vi "בדיקת מתח שחרור של סליל פיקוד ללא עומס 4.vi"(7 "resultUserPrompt":bool=TRUE, 8 "error":errorcluster, 11 "Path for Log":path) -> (0 "error out":errorcluster, 1 "מצב ממסר פתוח/סגור":bool, 2 "מתח פתיחת הממסר":dbl format="%.4f", 3 "מתח מוצא מהספק":dbl format="%.4f")   [LabVIEW 2015]
uses:
  <vilib>/DAQmx/write.llb/DAQmx Write (Digital Bool 1Line 1Point).vi
  <vilib>/DAQmx/create/channels.llb/DAQmx Create Channel (DO-Digital Output).vi
  <vilib>/DAQmx/miscellaneous.llb/DAQmx Fill In Error Info.vi
panel:
  out "progress":dbl(slide) scale=0.0..11.0
  out "error IO DMM":errorcluster
  in  "Stop Button":bool
  # "Right-Click to\nexplain error"
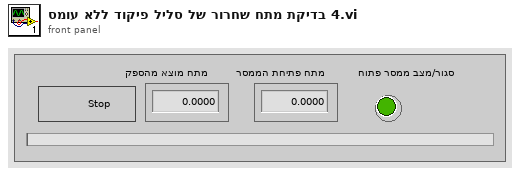
[diagram p1: front panel]
types:
  T1 = enum32{"Invalid", "Standard", "Closed", "Hidden", "Minimized", "Maximized"}
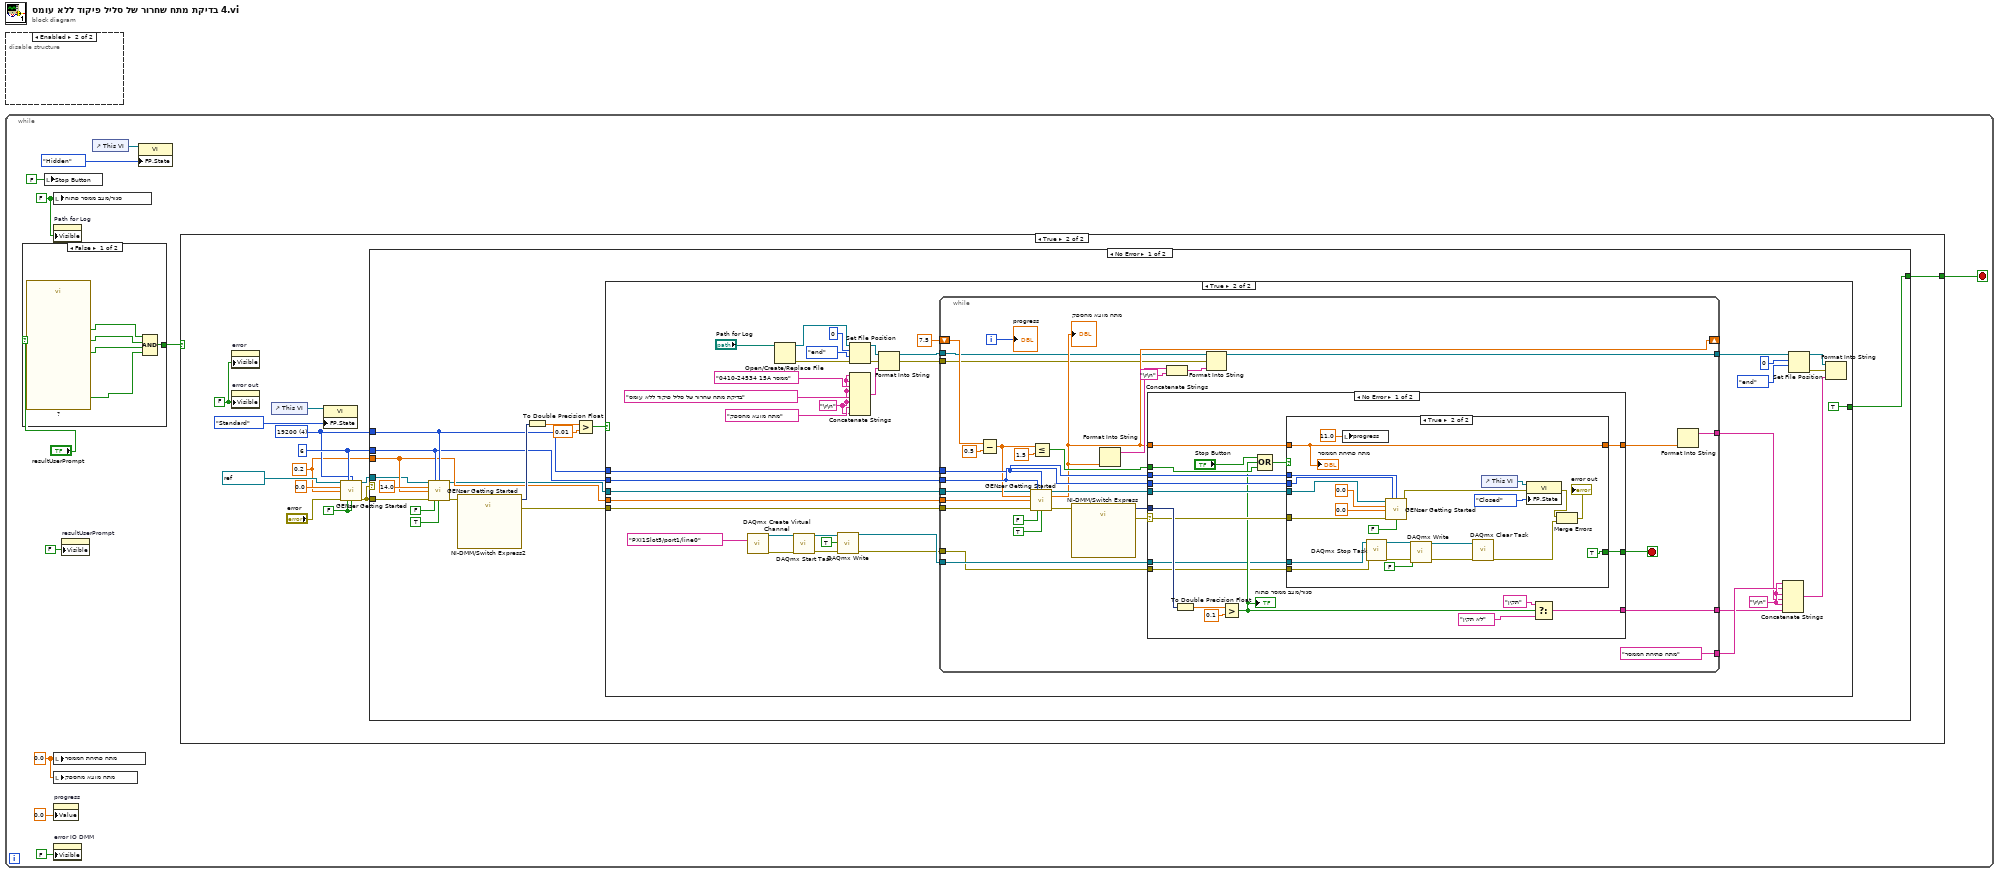
[diagram p0: block diagram]
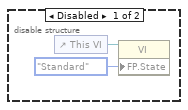
[diagram p2: hidden frame]
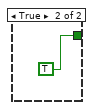
[diagram p3: hidden frame]
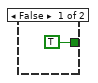
[diagram p4: hidden frame]
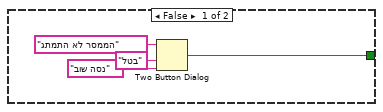
[diagram p5: hidden frame]
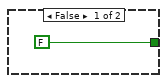
[diagram p6: hidden frame]
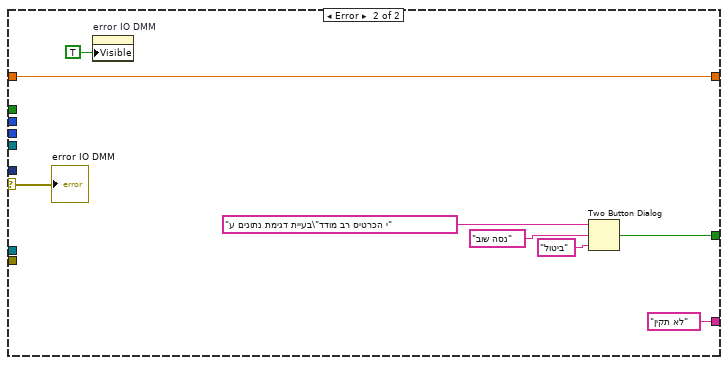
[diagram p7: hidden frame]
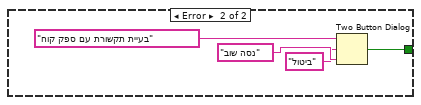
[diagram p8: hidden frame]
diagram:
  n1 = disable-structure shown="Enabled" {
    frame Disabled {
      n2 = control-ref of="This VI"() -> (w1:refnum<vi>)
      n3 = property class="VI"(reference=w1, "FP.State"=T1."Standard" ("Front Panel Window:State")) -> ()  [unwired: 1 in, 2 out]
    }
    frame Enabled {
    }
  }
  n4 = while {
    stop <- w3 stop-if-true
    w7 = FALSE ("מגע סגור")
    w10 = 0.0 ("signals out")
    n5 = case shown="False" "resultUserPrompt" {
      tunnel: [w18 TRUE] -> w4
      frame False {
        n6 = call "?"() -> ("הדקי הרב מודד"=w14:bool, "(מגע שלילי (מעטפת"=w15:bool, "A מגע חיובי"=w16:bool, "OK"=w17:bool)  [unwired: 15 in, 1 out]
        n7 = Compound Arithmetic op=AND(w17, w16, w15, w14) -> (w18:bool)
      }
      frame True {
      }
    }
    n8 = local write "Stop Button"(FALSE ("Reset (T)")) -> ()
    n9 = local write "מצב ממסר פתוח/סגור"(w7) -> ()
    n10 = property on="Path for Log" class="Path"("Visible"=w7) -> ()  [unwired: 2 in, 2 out]
    n11 = local write "מתח פתיחת הממסר"(w10) -> ()
    n12 = local write "מתח מוצא מהספק"(w10) -> ()
    n13 = property on="progress" class="Slide (strict)"("Value"=0.0 ("progress")) -> ()  [unwired: 2 in, 2 out]
    n14 = property on="error IO DMM" class="Clust (strict)"("Visible"=FALSE) -> ()  [unwired: 2 in, 2 out]
    n15 = property on="resultUserPrompt" class="Bool (strict)"("Visible"=FALSE) -> ()  [unwired: 2 in, 2 out]
    n16 = control-ref of="This VI"() -> (w9:refnum<vi>)
    n17 = property class="VI"(reference=w9, "FP.State"=T1."Hidden" ("Front Panel Window:State")) -> ()  [unwired: 1 in, 2 out]
    n18 = case shown="True" w4 {
      tunnel: [TRUE ("T button?") w25] -> w3
      frame False {
      }
      frame True {
        w23 = FALSE ("Visible")
        w24 = FALSE ("Output On (T)")
        w29 = u16 4 items=["1200", "2400", "4800", "9600", "19200"] ("BAUD")
        w30 = i16 6 ("GEN Addr")
        w26 = 0.2 ("Current Limit")
        n19 = property on="error" class="Clust (strict)"("Visible"=w23) -> ()  [unwired: 2 in, 2 out]
        n20 = property on="error out" class="Clust (strict)"("Visible"=w23) -> ()  [unwired: 2 in, 2 out]
        n21 = control-ref of="This VI"() -> (w21:refnum<vi>)
        n22 = property class="VI"(reference=w21, "FP.State"=T1."Standard" ("Front Panel Window:State")) -> ()  [unwired: 1 in, 2 out]
        n23 = call "GENser Getting Started.vi"("VISA"=refnum<visa-resource-name> "COM6", "GEN Addr"=w30, "BAUD"=w29, "Voltage Limit"=0.0, "Current Limit"=w26, "error"="error", "Reset (T)"=w24, "Output On (T)"=w24) -> ("VISA out"=w31:refnum<visa-resource-name>, "error out"=w32:errorcluster)  [unwired: 4 in, 2 out]
        n24 = case shown="No Error" w32 {
          tunnel: w32 -> [w42 _]
          tunnel: w31 -> [w38 _]
          tunnel: w30 -> [w40 _]
          tunnel: w29 -> [w41 _]
          tunnel: w26 -> [w39 _]
          tunnel: [w34 w177] -> w25
          frame No Error {
            n25 = call "GENser Getting Started.vi"("VISA"=w38, "GEN Addr"=w40, "BAUD"=w41, "Voltage Limit"=14.0, "Current Limit"=w39, "error"=w42, "Reset (T)"=FALSE, "Output On (T)"=TRUE) -> ("VISA out"=w37:refnum<visa-resource-name>, "error out"=w46:errorcluster)  [unwired: 4 in, 2 out]
            n26 = call "NI-DMM/Switch Express2"("error in"=w46) -> ("signals out"=w45:dynamicdata, "error out"=w43:errorcluster)  [unwired: 16 in, 1 out]
            n27 = To Double Precision Float(number=w45) -> (double precision float=w36:dbl)
            n28 = Greater?(x=w36, y=0.01) -> (0:w44:bool)
            n29 = case shown="True" w44 {
              tunnel: w43 -> [_ w92]
              tunnel: w40 -> [_ w91]
              tunnel: w41 -> [_ w90]
              tunnel: w39 -> [_ w89]
              tunnel: w37 -> [_ w87]
              tunnel: [w50 TRUE] -> w34
              frame False {
                n30 = Two Button Dialog(message="הממסר לא התמתג", 1:"נסה שוב" ("T button name (\"OK\")"), 2:"בטל" ("T button name (\"OK\")")) -> (T button?=w50:bool)
              }
              frame True {
                w63 = "\r\n"
                w86 = "\r\n"
                n31 = call-poly <vilib>:"DAQmx Create Virtual Channel.vi"("lines"=tag "PXI1Slot5/port1/line0") -> ("task out"=w61:refnum<k21>, "error out"=w62:errorcluster)  [unwired: 13 in]
                n32 = Open/Create/Replace File(file path (use dialog)="Path for Log") -> (refnum out=w74:refnum<file>, error out=w73:errorcluster)  [unwired: 5 in, 1 out]
                n33 = call <vilib>:"DAQmx Start Task.vi"("task/channels in"=w61, "error in"=w62) -> ("task out"=w59:refnum<k21>, "error out"=w58:errorcluster)  [unwired: 12 in]
                n34 = call-poly <vilib>:"DAQmx Write.vi"("task/channels in"=w59, "data"=TRUE, "error in"=w58) -> ("task out"=w56:refnum<k21>, "error out"=w55:errorcluster)  [unwired: 10 in, 1 out]
                n35 = Set File Position(offset (in bytes) (0)=i64 0, refnum=w74, from (0:start)=enum16{"start", "end", "current"}."end", error in=w73) -> (refnum out=w69:refnum<file>, error out=w64:errorcluster)
                n36 = Concatenate Strings(w63, w63, "0410-24534 15A ממסר", w63, "בדיקת מתח שחרור של סליל פיקוד ללא עומס", w63, "מתח מוצא מהספק", w63) -> (w72:string)
                n37 = Format Into String(initial string=w69, error in=w64, w72) -> (resulting string=w66:refnum<file>, error out=w65:errorcluster)  [unwired: 1 in]
                n38 = while {
                  tunnel: w92 -> [w123]
                  tunnel: w91 -> [w115]
                  tunnel: w90 -> [w114]
                  tunnel: w89 -> [w121]
                  shift-right: [w97] -> _
                  shift-left: 7.5 ("y") -> [w119]
                  tunnel: w87 -> [w107]
                  tunnel: [w102] -> w81
                  tunnel: ["מתח פתיחת הממסר"] -> w80
                  tunnel: [w100] -> w79
                  tunnel: [w99] -> w78
                  tunnel: w66 -> [w96]
                  tunnel: w65 -> [w95]
                  tunnel: w56 -> [w94]
                  tunnel: w55 -> [w93]
                  i -> [w108]
                  stop <- w116 stop-if-true
                  n39 = Subtract(x=w119, y=0.5) -> (x-y=w111:dbl)
                  n40 = call "GENser Getting Started.vi"("VISA"=w107, "GEN Addr"=w115, "BAUD"=w114, "Voltage Limit"=w111, "Current Limit"=w121, "error"=w123, "Reset (T)"=FALSE, "Output On (T)"=TRUE) -> ("VISA out"=w113:refnum<visa-resource-name>, "Output Voltage"=w97:dbl, "error out"=w118:errorcluster)  [unwired: 4 in, 1 out]
                  "מתח מוצא מהספק" <- w97
                  n41 = Less Or Equal?(x=w111, y=1.5) -> (x <= y?=w110:bool)
                  n42 = call "NI-DMM/Switch Express"("error in"=w118) -> ("signals out"=w117:dynamicdata, "error out"=w109:errorcluster)  [unwired: 16 in, 1 out]
                  n43 = Format Into String(w97) -> (resulting string=w104:string)  [unwired: 3 in, 1 out]
                  n44 = case shown="No Error" w109 {
                    selector: w109 -> [w133 w174]
                    tunnel: w117 -> [w142 _]
                    tunnel: [w139 w170] -> w116
                    tunnel: w115 -> [w138 _]
                    tunnel: w114 -> [w137 _]
                    tunnel: w113 -> [w136 _]
                    tunnel: w110 -> [w135 _]
                    tunnel: w97 -> [w134 w168]
                    tunnel: [w127 w168] -> w103
                    tunnel: [w126 "לא תקין"] -> w99
                    tunnel: w94 -> [w125 _]
                    tunnel: w93 -> [w124 _]
                    frame No Error {
                      n45 = To Double Precision Float(number=w142) -> (double precision float=w132:dbl)
                      n46 = Greater?(x=w132, y=0.1) -> (0:w128:bool)
                      "מצב ממסר פתוח/סגור" <- w128
                      n47 = Compound Arithmetic op=OR("Stop Button", w128, w135) -> (w141:bool)
                      n48 = case shown="True" w141 {
                        tunnel: [FALSE TRUE] -> w139
                        tunnel: w138 -> [_ w165]
                        tunnel: w137 -> [_ w164]
                        tunnel: w136 -> [_ w163]
                        tunnel: w133 -> [_ w160]
                        tunnel: w134 -> [_ w154]
                        tunnel: [_ w154] -> w127
                        tunnel: w125 -> [_ w148]
                        tunnel: w124 -> [_ w147]
                        frame False {
                        }
                        frame True {
                          n49 = local write "progress"(11.0 ("progress")) -> ()
                          n50 = call <vilib>:"DAQmx Stop Task.vi"("task/channels in"=w148, "error in"=w147) -> ("task out"=w153:refnum<k21>, "error out"=w152:errorcluster)  [unwired: 12 in]
                          n51 = call "GENser Getting Started.vi"("VISA"=w163, "GEN Addr"=w165, "BAUD"=w164, "Voltage Limit"=0.0, "Current Limit"=0.0, "error"=w160, "Output On (T)"=FALSE) -> ("error out"=w155:errorcluster)  [unwired: 5 in, 3 out]
                          n52 = call-poly <vilib>:"DAQmx Write.vi"("task/channels in"=w153, "data"=FALSE, "error in"=w152) -> ("task out"=w151:refnum<k21>, "error out"=w150:errorcluster)  [unwired: 10 in, 1 out]
                          n53 = call <vilib>:"DAQmx Clear Task.vi"("task in"=w151, "error in"=w150) -> ("error out"=w146:errorcluster)  [unwired: 13 in]
                          n54 = control-ref of="This VI"() -> (w156:refnum<vi>)
                          n55 = property class="VI"(reference=w156, error in=w155, "FP.State"=T1."Closed" ("Front Panel Window:State")) -> (error out=w145:errorcluster)  [unwired: 1 out]
                          n56 = Merge Errors(w145, w146) -> (→"error out":errorcluster)
                          "מתח פתיחת הממסר" <- w154
                        }
                      }
                      n57 = Select(t="תקין", s=w128, f="לא תקין") -> (s? t:f=w126:string)
                    }
                    frame Error {
                      n58 = property on="error IO DMM" class="Clust (strict)"("Visible"=TRUE) -> ()  [unwired: 2 in, 2 out]
                      n59 = Two Button Dialog(message="בעיית דגימת נתונים ע\"י הכרטיס רב מודד", 1:"ביטול" ("F button name (\"Cancel\")"), 2:"נסה שוב" ("T button name (\"OK\")")) -> (T button?=w170:bool)
                      "error IO DMM" <- w174
                    }
                  }
                  n60 = Concatenate Strings(w104, "\r\n") -> (w98:string)
                  n61 = Format Into String(initial string=w96, error in=w95, w98) -> (resulting string=w102:refnum<file>)  [unwired: 1 in, 1 out]
                  n62 = Format Into String(w103) -> (resulting string=w100:string)  [unwired: 3 in, 1 out]
                  "progress" <- w108
                }
                n63 = Concatenate Strings(w86, w80, w86, w79, w86, w78) -> (w77:string)
                n64 = Set File Position(offset (in bytes) (0)=i64 0, refnum=w81, from (0:start)=enum16{"start", "end", "current"}."end") -> (refnum out=w83:refnum<file>, error out=w82:errorcluster)  [unwired: 1 in]
                n65 = Format Into String(initial string=w83, error in=w82, w77) -> ()  [unwired: 1 in, 2 out]
              }
            }
          }
          frame Error {
            n66 = Two Button Dialog(message="בעיית תקשורת עם ספק קוח", 1:"נסה שוב" ("T button name (\"OK\")"), 2:"ביטול" ("F button name (\"Cancel\")")) -> (T button?=w177:bool)
          }
        }
      }
    }
  }
